vi "Read image_SR.vi"(7 "Concatenating string":string, 8 "error in (no error)":errorcluster, 9 "Read type":string(combo)="Direct read", 10 "Filepath type":string(combo)="Read from separate files", 11 "Image filepath array":path[](array[path])) -> (0 "error out":errorcluster, 2 "Image names":string[](array[string]), 3 "Image \narray":T1[](array[typedef]))   [LabVIEW 2019]
uses:
  <vilib>/vision/Image Controls.llb/IMAQ Image.ctl
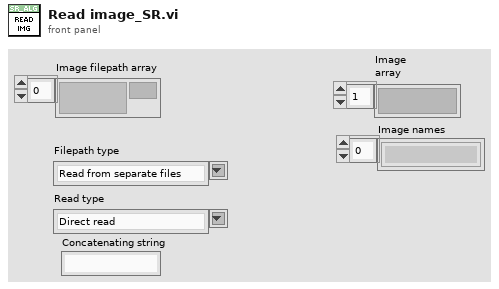
[diagram p1: front panel]
types:
  T1 = typedef "IMAQ Image.ctl" = refnum<image>
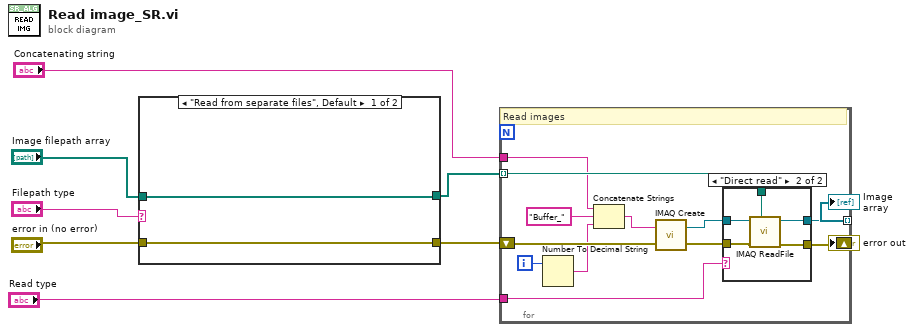
[diagram p0: block diagram]
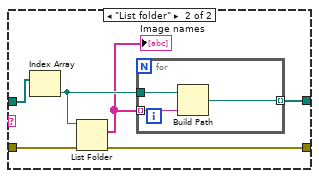
[diagram p2: hidden frame]
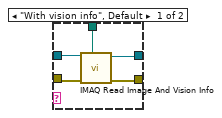
[diagram p3: hidden frame]
diagram:
  n1 = case shown="\"Read from separate files\", Default" "Filepath type" {
    tunnel: "Image filepath array" -> [w11 w17]
    tunnel: "error in (no error)" -> [w10 w16]
    tunnel: [w10 w14] -> w7
    tunnel: [w11 w13] -> w6
    frame "Read from separate files", Default {
    }
    frame "List folder" {
      n2 = Index Array(array=w17) -> (element=w15:path)  [unwired: 1 in]
      n3 = List Folder(path=w15, error in=w16) -> (filenames=w12:string[], error out=w14:errorcluster)  [unwired: 2 in, 2 out]
      "Image names" <- w12
      n4 = for {
        tunnel: w12 -> [w19] mode=indexing
        tunnel: w15 -> [w20]
        tunnel: [w18] -> w13 mode=indexing
        n5 = Build Path(base path=w20, name or relative path=w19) -> (appended path=w18:path)
      }
    }
  }
  n6 = for {
    shift-right: [w30] -> w4
    shift-left: w7 -> [w32]
    tunnel: w6 -> [w24] mode=indexing
    tunnel: [w23] -> w3 mode=indexing
    tunnel: "Read type" -> [w22]
    tunnel: "Concatenating string" -> [w21]
    i -> [w28]
    # "Read images"
    n7 = Number To Decimal String(number=w28) -> (decimal integer string=w26:string)  [unwired: 1 in]
    n8 = Concatenate Strings(w21, "Buffer_", w26) -> (w25:string)
    n9 = call "IMAQ Create"("Image Name"=w25, "error in (no error)"=w32) -> ("New Image"=w29:T1, "error out"=w31:errorcluster)  [unwired: 3 in]
    n10 = case shown="\"Direct read\"" w22 {
      tunnel: w31 -> [w36 w42]
      tunnel: [w35 w41] -> w30
      tunnel: w29 -> [w37 w40]
      tunnel: w24 -> [w33 w39]
      tunnel: [w34 w38] -> w23
      frame "With vision info", Default {
        n11 = call "IMAQ Read Image And Vision Info"("File Path"=w33, "error in (no error)"=w36, "Image"=w37) -> ("error out"=w35:errorcluster, "Image Out"=w34:T1)  [unwired: 6 in, 1 out]
      }
      frame "Direct read" {
        n12 = call "IMAQ ReadFile"("File Path"=w39, "error in (no error)"=w42, "Image"=w40) -> ("error out"=w41:errorcluster, "Image Out"=w38:T1)  [unwired: 4 in, 3 out]
      }
    }
  }
  "error out" <- w4
  "Image \narray" <- w3
